vi "CutWaveform(1CH).vi"(11 "Waveform in":waveform(sgl)) -> (3 "Waveform out":waveform(sgl))   [LabVIEW 2016, in "McsaAnalysisFunctions.lvlib"]
uses:
  <vilib>/addons/InsightCM/Utilities/Analysis/MCSA/McsaAnalysisFunctions.lvlib
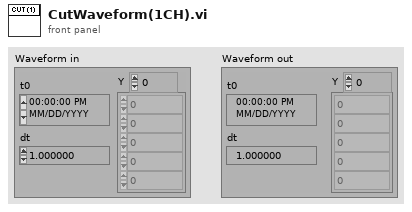
[diagram p1: front panel]
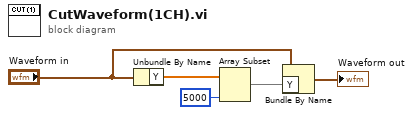
[diagram p0: block diagram]
diagram:
  n1 = Unbundle By Name("Waveform in") -> ("Y"=w2:sgl[])
  n2 = Array Subset(array=w2, length=5000) -> (w3:sgl[])  [unwired: 1 in]
  n3 = Bundle By Name(cluster="Waveform in", "Y"=w3) -> (→"Waveform out":waveform(sgl))
